vi "Project.vi"() -> ()   [LabVIEW 2026]
doc: "This example performs writes and reads on a serial port, as directed by the user. You can press the Write and Read buttons, and change the Read Count, while the example is running.\n\nThe parameters set for the serial port must match the parameters of the connected instrument or device. In this example, the Read Count parameter specifies the number of bytes that the serial port reads. If there were more bytes at the port than the specified number, those bytes would not be read. If there were less bytes at the port than the specified number, you would receive a timeout error.\n\nThis example expands upon the flow control options for XON and XOFF, allowing the user to choose those control characters. Also, the user can enable or disable a termination character. Some devices require a termination character in order to identify the end of command strings. Some devices send a termination character to signify the end of data to be read. This example shows how you can end the Read operation once a termination character is detected in the buffer and/or append a termination character at the end of the Write data."
uses:
  Serial - Settings.ctl
  Control 1.ctl
  ESP32-PSOC-State Machine-1.ctl
  <vilib>/Instr/_visa.llb/VISA Flush IO Buffer Mask.ctl
  <vilib>/Instr/_visa.llb/VISA Configure Serial Port (Instr).vi
panel:
  in  "HARD START":bool
  in  "INTERMEDIATE START":bool
  out "error":bool
  out "Connected":bool
  out "Serial Settings:Number of Bytes at Serial Port":u32
  out "Processing":string
  in  "EASY START":bool
  in  "IDENTIFY":bool
  in  "CALIBRATE":bool
  in  "Enum":T1
  in  "Termination Character":u8=10 format="%.0x"
  in  "End Write on Termination Character?":bool=TRUE
  in  "EXIT":bool
  out "Read Count":u32=1000
  out "Raw Response":string
  in  "XON/XOFF Characters":T2={"XON"=enum."DC1", "XOFF"=enum."DC3"}
  in  "Serial Settings":T3={"baud rate"=115200, "data bits"=8, "parity"=enum."None", "stop bits"=10, "flow control"=0} {"flow control" items=["None"=0, "XON/XOFF"=1, "RTS/CTS"=2, "DTR/DSR"=4]; "stop bits" items=["1.0"=10, "1.5"=15, "2.0"=20]; "data bits" min=5 max=8 step=1; "baud rate" items=["75"=75, "110"=110, "134"=134, "150"=150, "300"=300, "600"=600, "1200"=1200, "1800"=1800, "2400"=2400, "4800"=4800, "7200"=7200, "9600"=9600, "14400"=14400, "19200"=19200, "28800"=28800, "38400"=38400, "56000"=56000, "57600"=57600, "115200"=115200, "128000"=128000, "230400"=230400]}
  in  "End Read on Termination Character?":bool=TRUE
  in  "Serial Port":refnum<visa-resource-name>="COM4"
  # "What is LabView currently doing?"
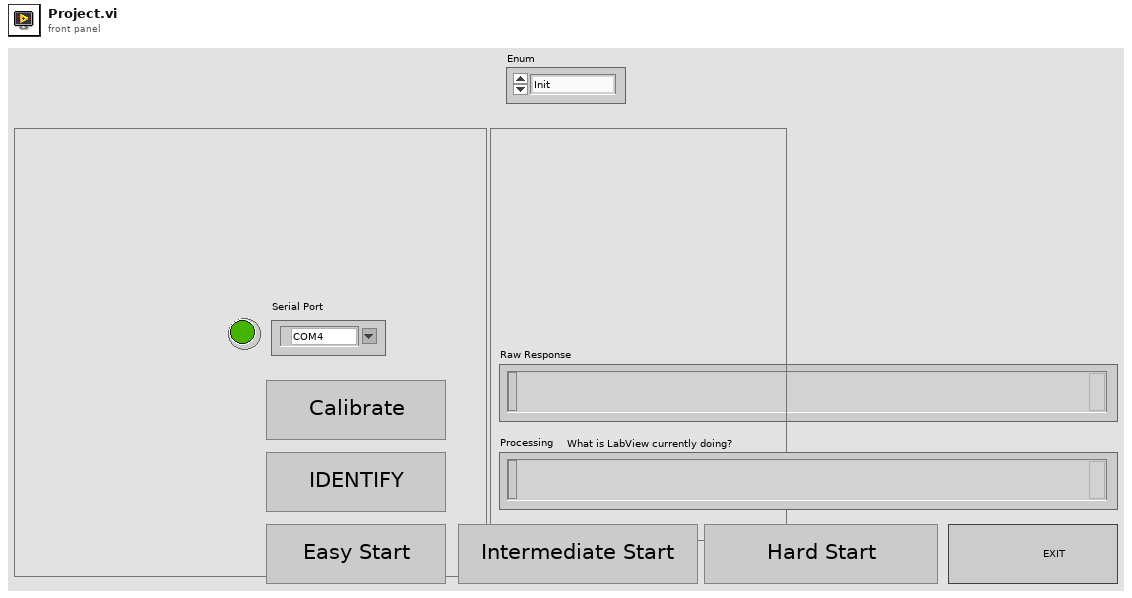
[diagram p1: front panel]
types:
  T1 = typedef "ESP32-PSOC-State Machine-1.ctl" = enum8{"Init", "Connect", "idle", "send", "wait", "receive", "que", "error", "exit"}
  T2 = typedef "Control 1.ctl" = cluster{"XON":enum16{"NUL", "SOH", "STX", "ETX", "EOT", "ENQ", "ACK", "BEL", "BS", "HT", "LF", "VT", "FF", "CR", "SO", "SI", "DLE", "DC1", "DC2", "DC3", "DC4", "NAK", "SYN", "ETB", "CAN", "EM", "SUB", "ESC", "FS", "GS", "RS", "US", "SP", "!", "\"", "#", "$", "%", "&", "'", "(", ")", "*", "+", ",", "- (-)", ".", "/", "0", "1", "2", "3", "4", "5", "6", "7", "8", "9", ":", ";", "<", "=", ">", "?", "@", "A", "B", "C", "D", "E", "F", "G", "H", "I", "J", "K", "L", "M", "N", "O", "P", "Q", "R", "S", "T", "U", "V", "W", "X", "Y", "Z", "[", "\\", "]", "^", "_", "`", "a", "b", "c", "d", "e", "f", "g", "h", "i", "j", "k", "l", "m", "n", "o", "p", "q", "r", "s", "t", "u", "v", "w", "x", "y", "z", "{", "|", "}", "~"}, "XOFF":enum16{"NUL", "SOH", "STX", "ETX", "EOT", "ENQ", "ACK", "BEL", "BS", "HT", "LF", "VT", "FF", "CR", "SO", "SI", "DLE", "DC1", "DC2", "DC3", "DC4", "NAK", "SYN", "ETB", "CAN", "EM", "SUB", "ESC", "FS", "GS", "RS", "US", "SP", "!", "\"", "#", "$", "%", "&", "'", "(", ")", "*", "+", ",", "- (-)", ".", "/", "0", "1", "2", "3", "4", "5", "6", "7", "8", "9", ":", ";", "<", "=", ">", "?", "@", "A", "B", "C", "D", "E", "F", "G", "H", "I", "J", "K", "L", "M", "N", "O", "P", "Q", "R", "S", "T", "U", "V", "W", "X", "Y", "Z", "[", "\\", "]", "^", "_", "`", "a", "b", "c", "d", "e", "f", "g", "h", "i", "j", "k", "l", "m", "n", "o", "p", "q", "r", "s", "t", "u", "v", "w", "x", "y", "z", "{", "|", "}", "~"}}
  T3 = typedef "Serial - Settings.ctl" = cluster{"baud rate":u32, "data bits":u16, "parity":enum16{"None", "Odd", "Even", "Mark", "Space"}, "stop bits":u16, "flow control":u16}
  T4 = enum16{"NUL", "SOH", "STX", "ETX", "EOT", "ENQ", "ACK", "BEL", "BS", "HT", "LF", "VT", "FF", "CR", "SO", "SI", "DLE", "DC1", "DC2", "DC3", "DC4", "NAK", "SYN", "ETB", "CAN", "EM", "SUB", "ESC", "FS", "GS", "RS", "US", "SP", "!", "\"", "#", "$", "%", "&", "'", "(", ")", "*", "+", ",", "- (-)", ".", "/", "0", "1", "2", "3", "4", "5", "6", "7", "8", "9", ":", ";", "<", "=", ">", "?", "@", "A", "B", "C", "D", "E", "F", "G", "H", "I", "J", "K", "L", "M", "N", "O", "P", "Q", "R", "S", "T", "U", "V", "W", "X", "Y", "Z", "[", "\\", "]", "^", "_", "`", "a", "b", "c", "d", "e", "f", "g", "h", "i", "j", "k", "l", "m", "n", "o", "p", "q", "r", "s", "t", "u", "v", "w", "x", "y", "z", "{", "|", "}", "~"}
  T5 = typedef "VISA Flush IO Buffer Mask.ctl" = u16
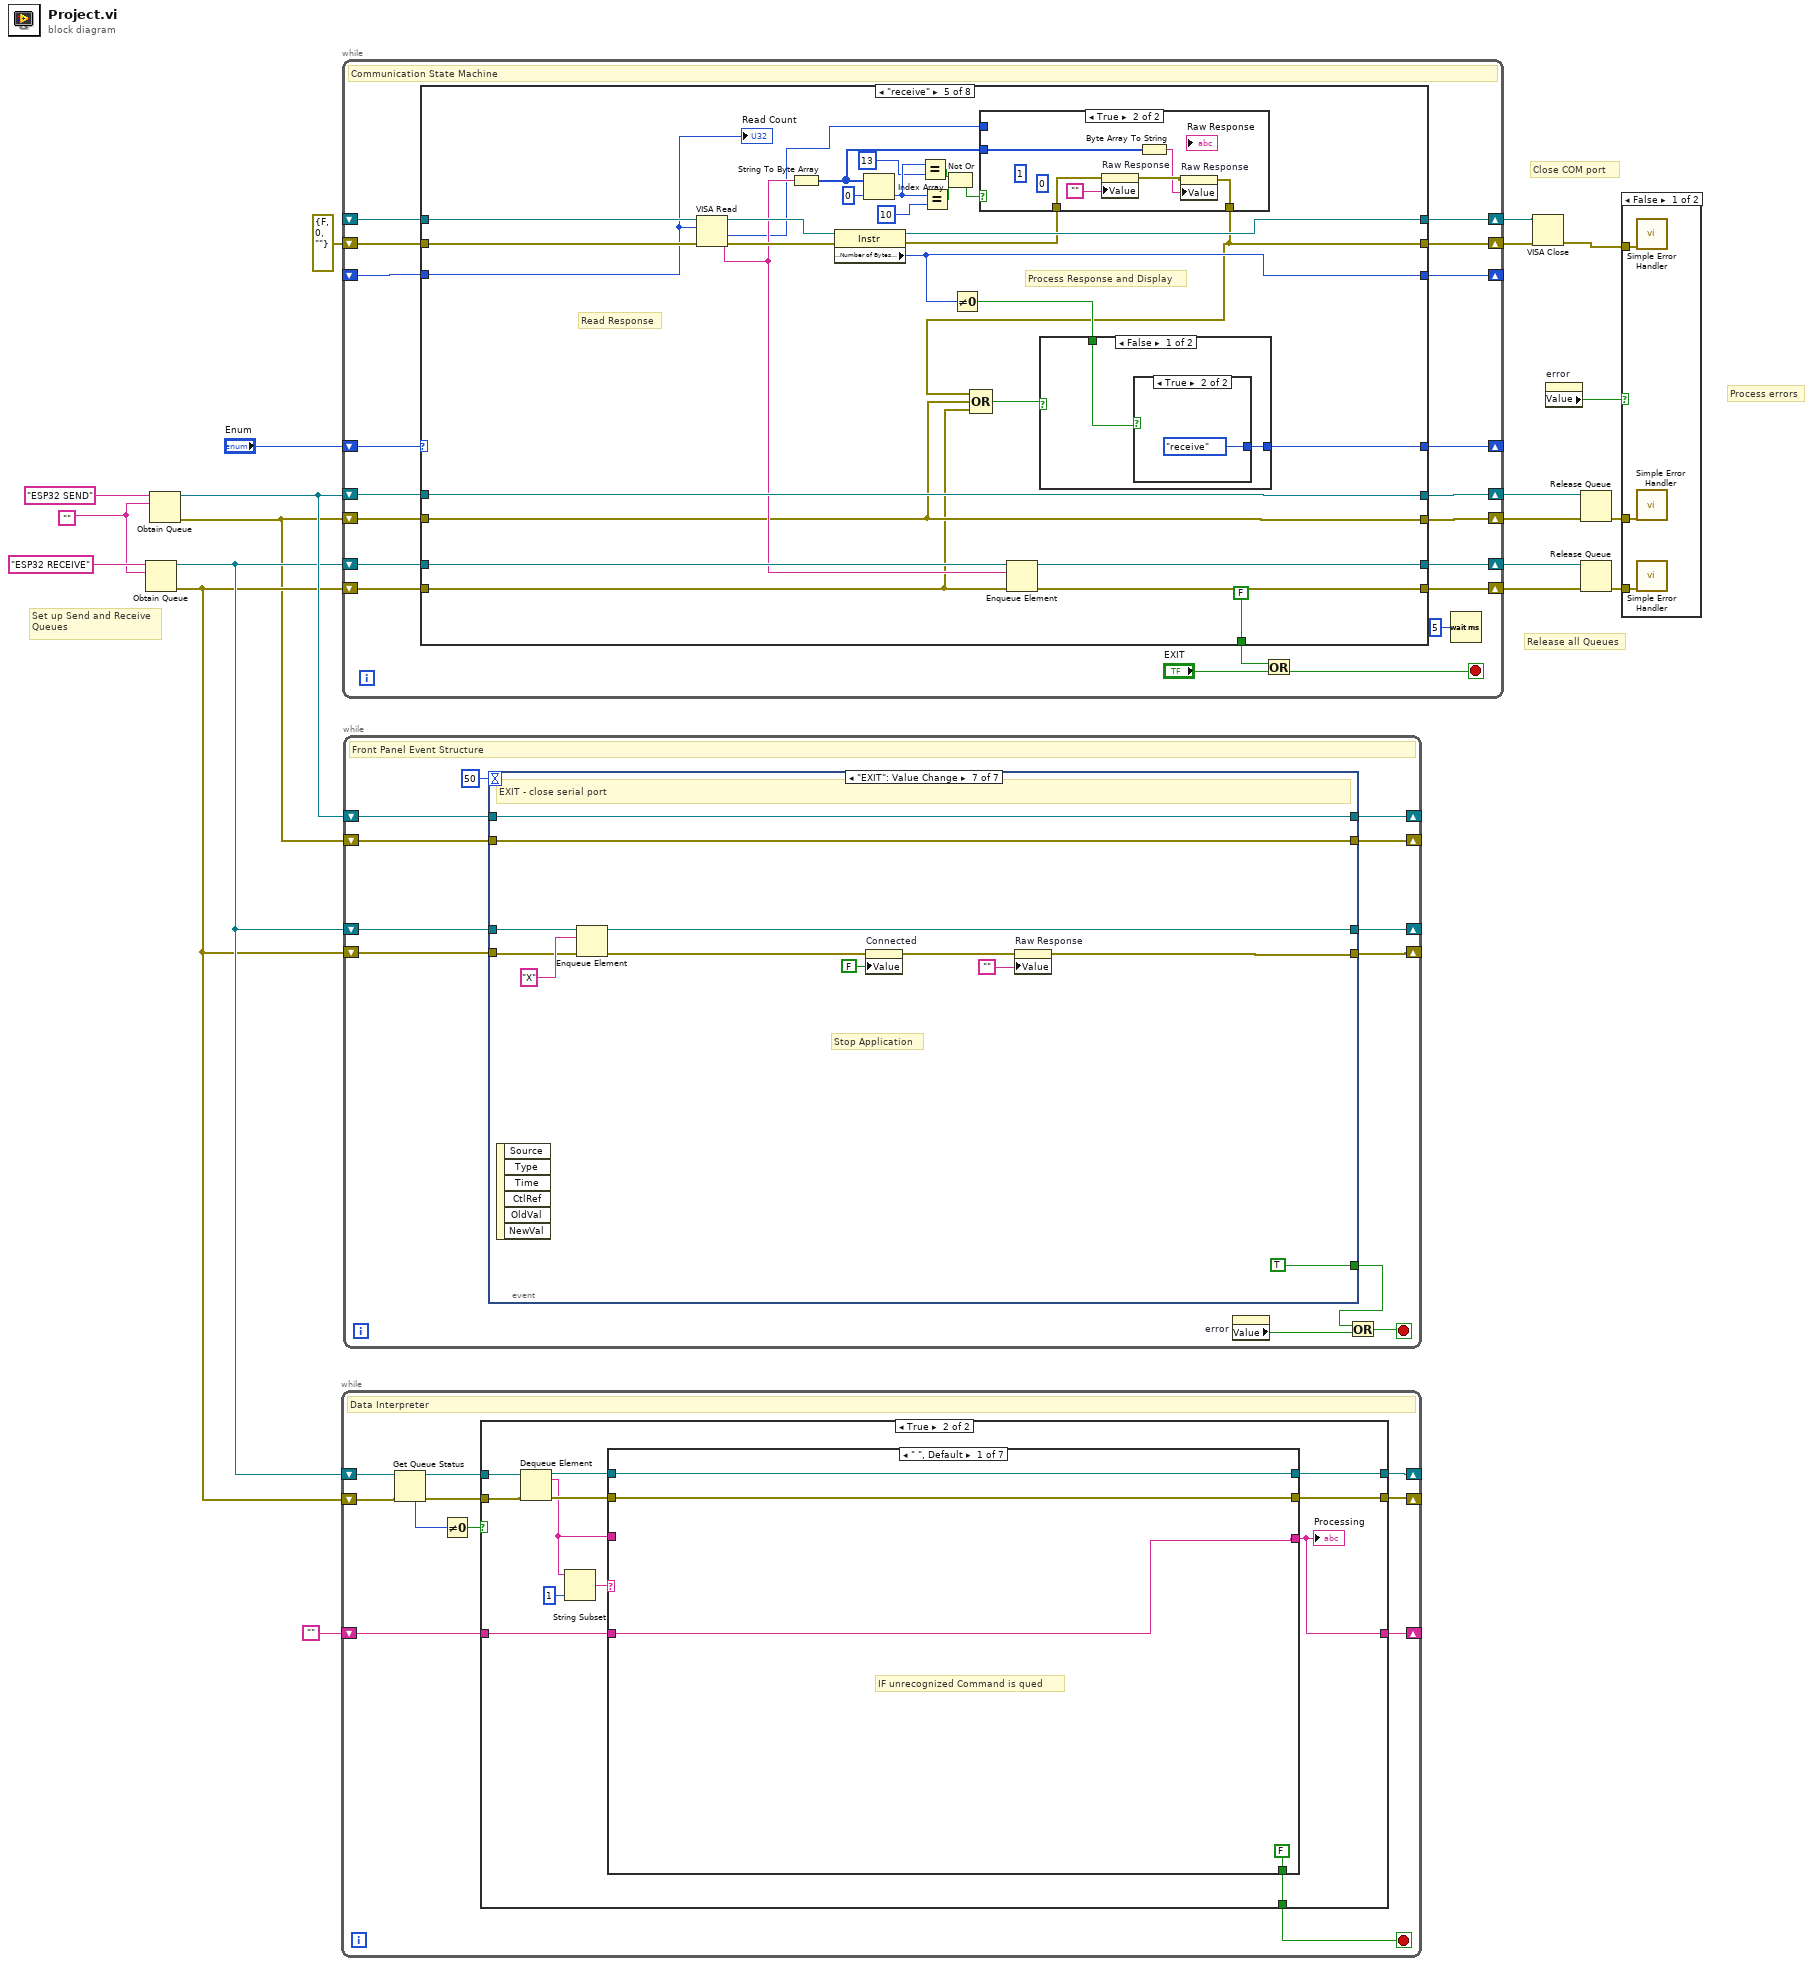
[diagram p0: block diagram]
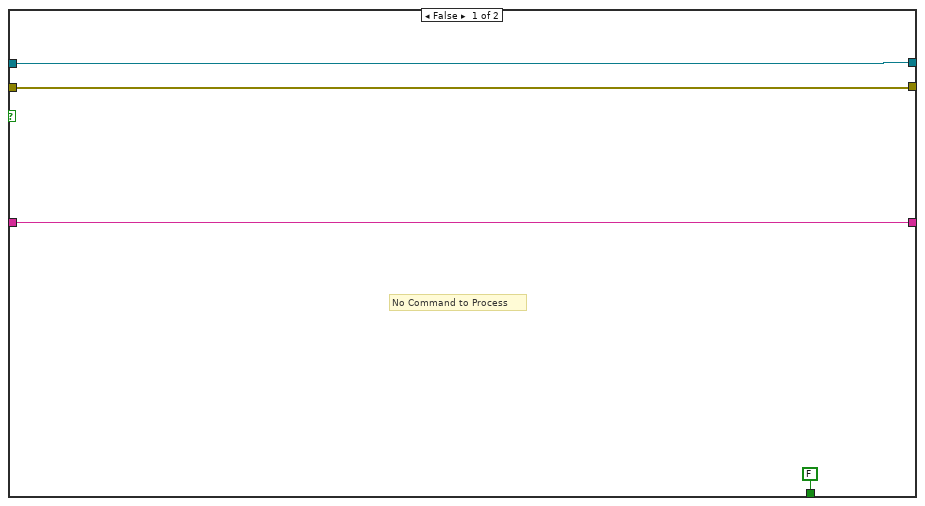
[diagram p3: hidden frame]
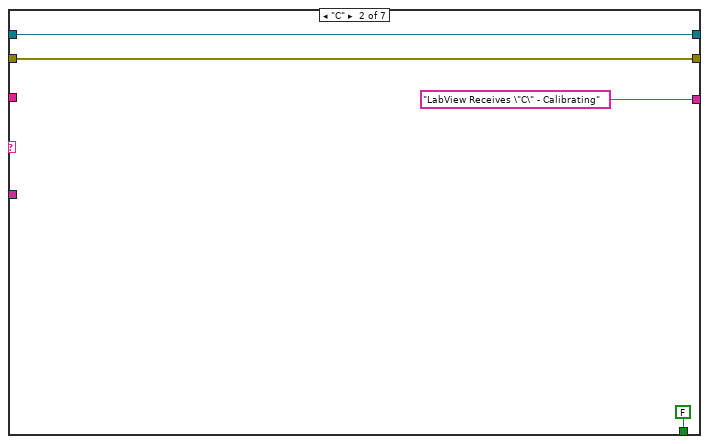
[diagram p4: hidden frame]
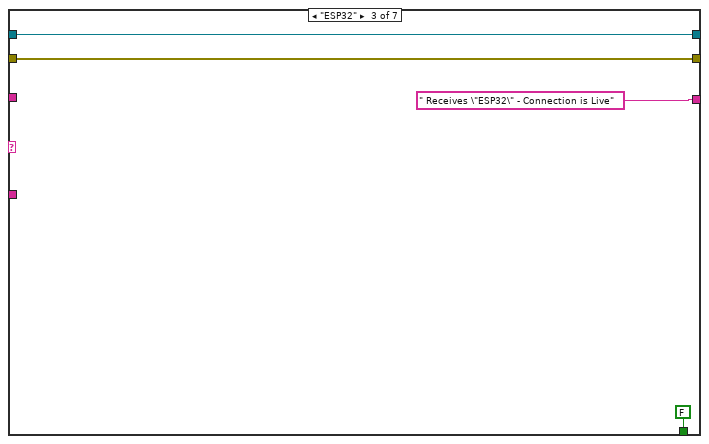
[diagram p5: hidden frame]
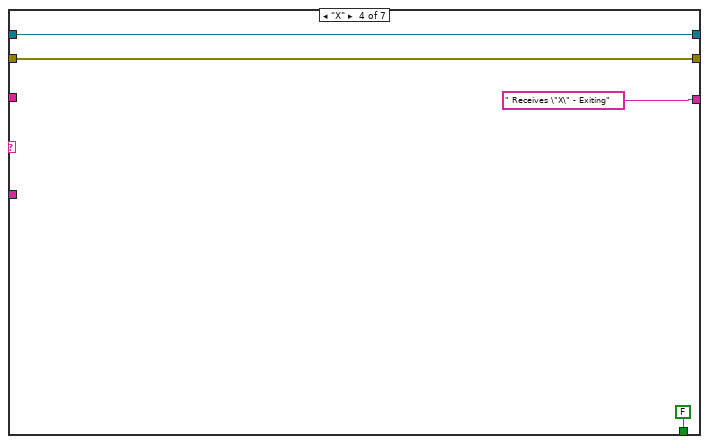
[diagram p6: hidden frame]
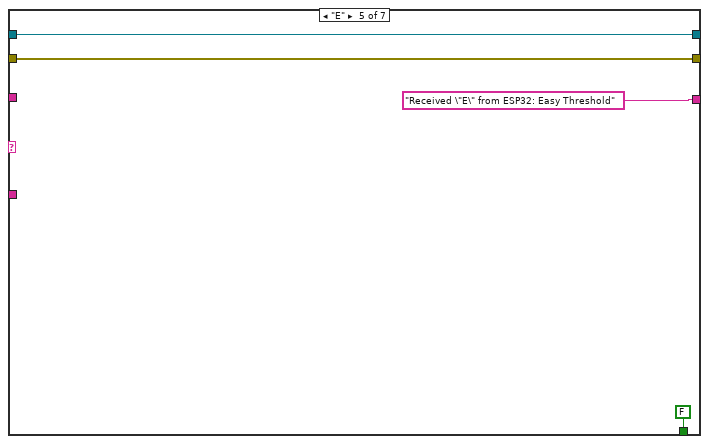
[diagram p7: hidden frame]
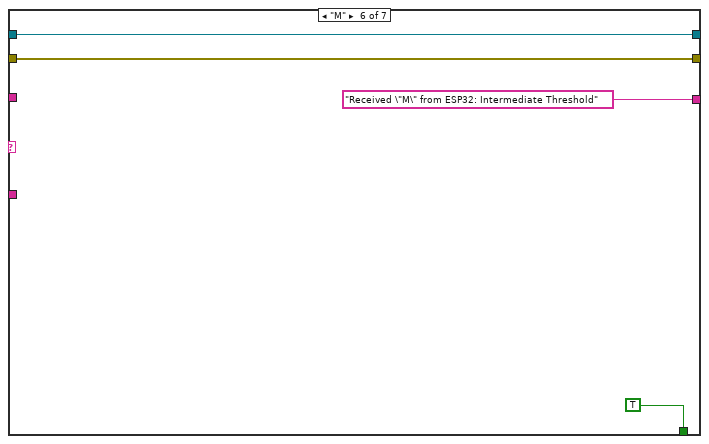
[diagram p8: hidden frame]
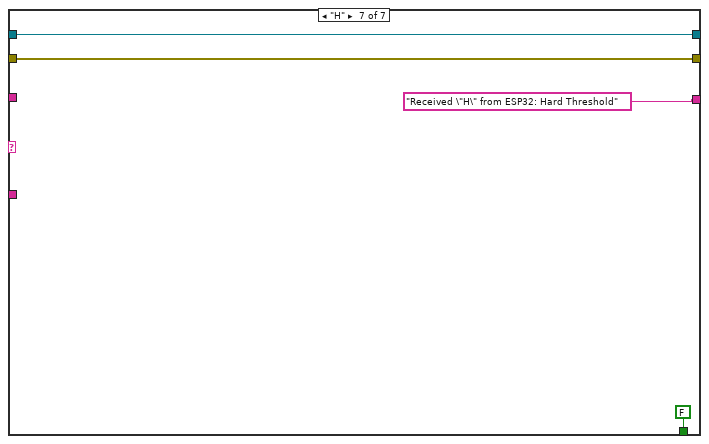
[diagram p9: hidden frame]
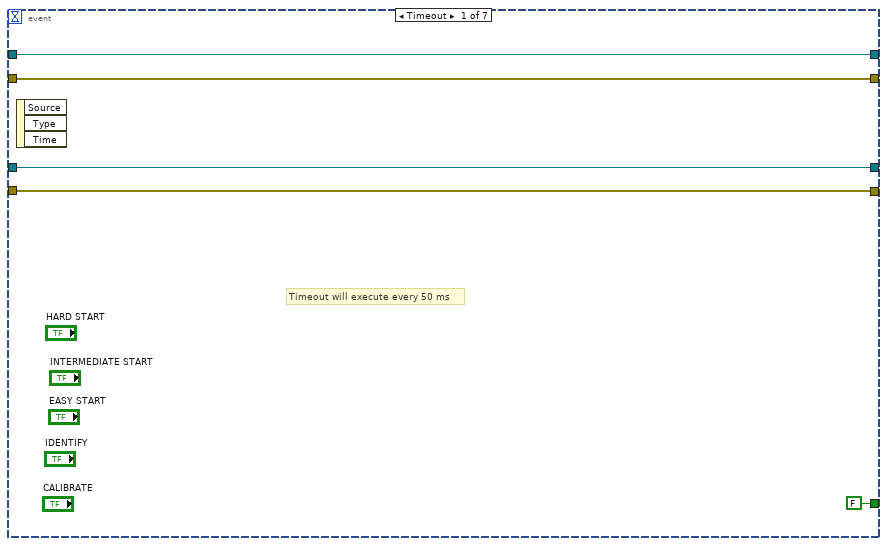
[diagram p10: hidden frame]
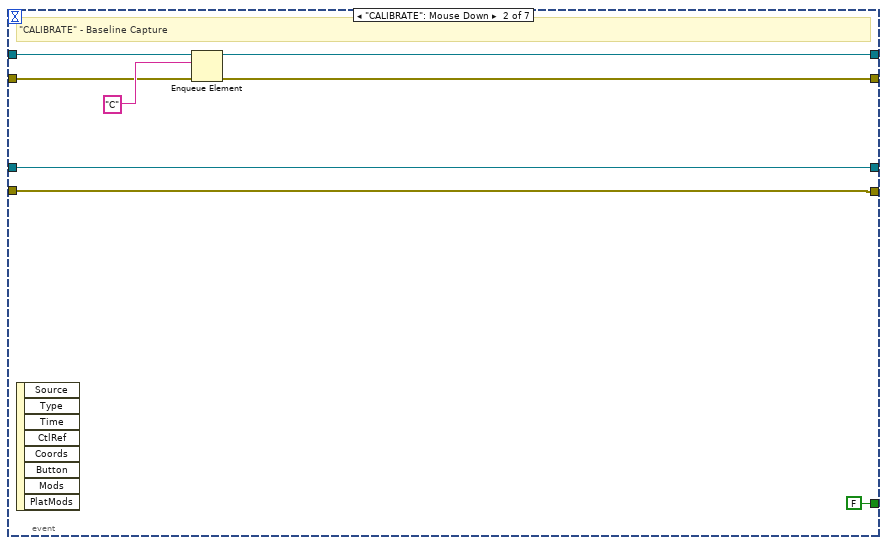
[diagram p11: hidden frame]
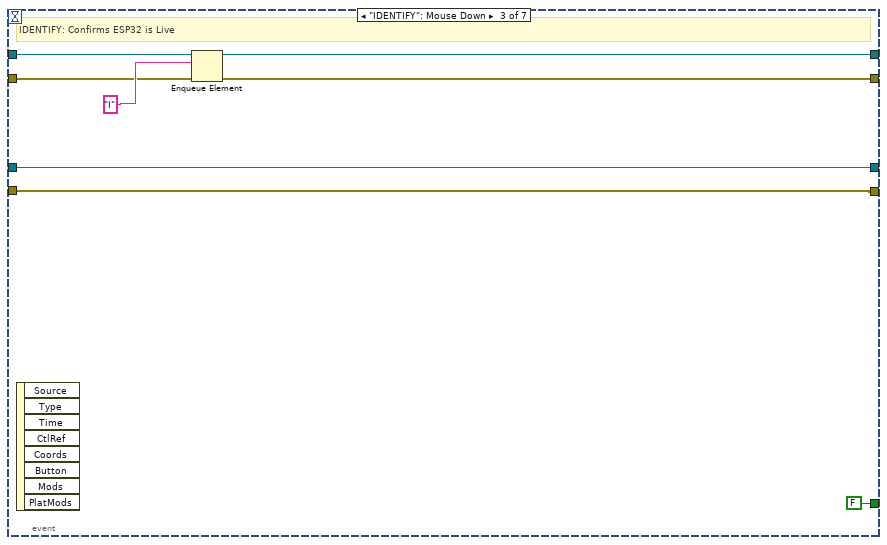
[diagram p12: hidden frame]
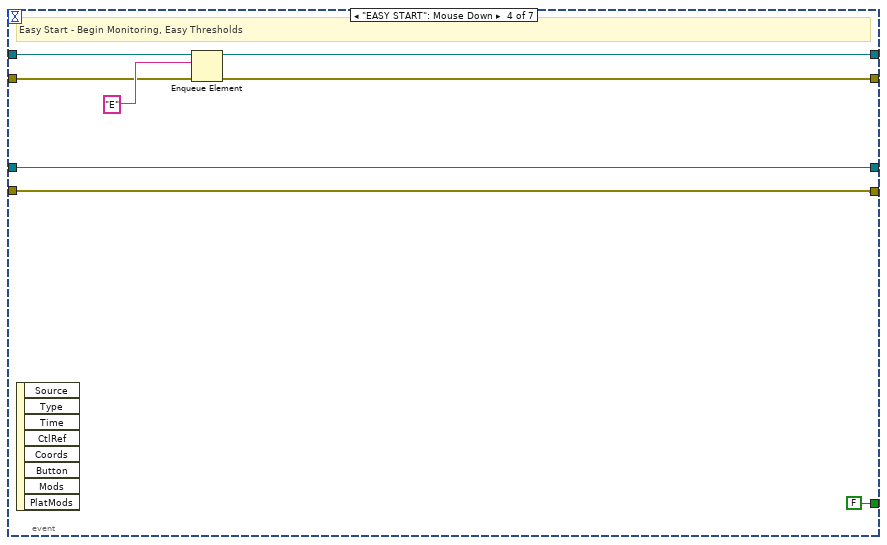
[diagram p13: hidden frame]
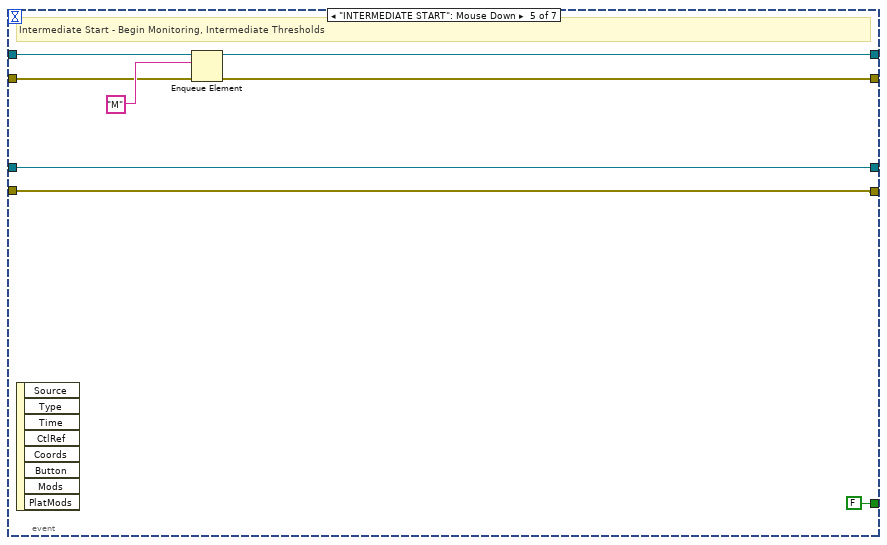
[diagram p14: hidden frame]
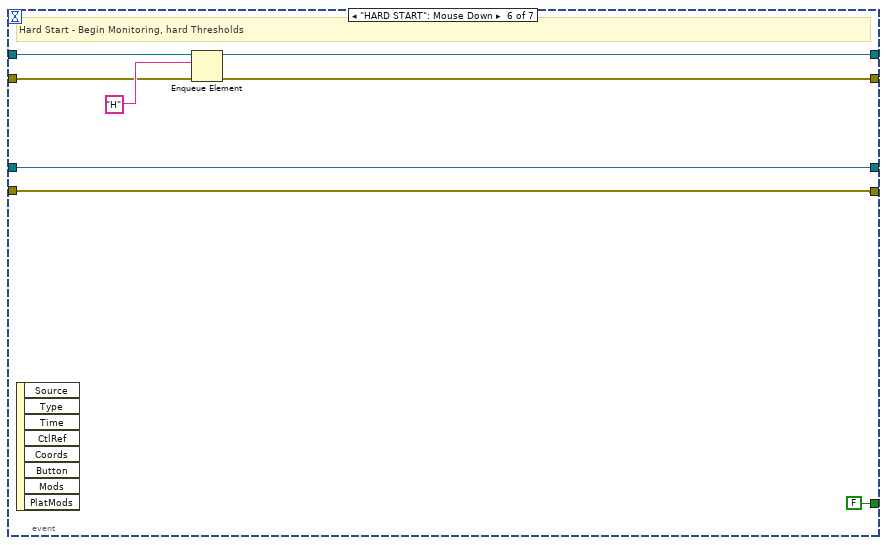
[diagram p15: hidden frame]
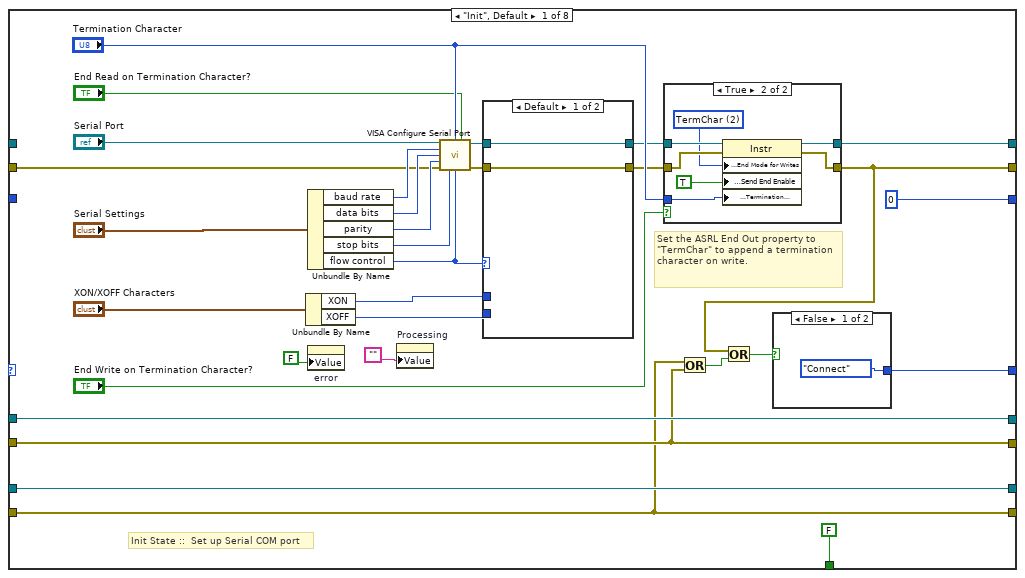
[diagram p16: hidden frame]
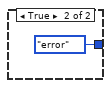
[diagram p17: hidden frame]
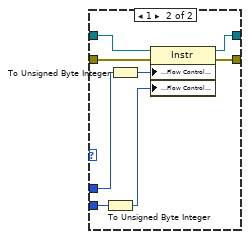
[diagram p19: hidden frame]
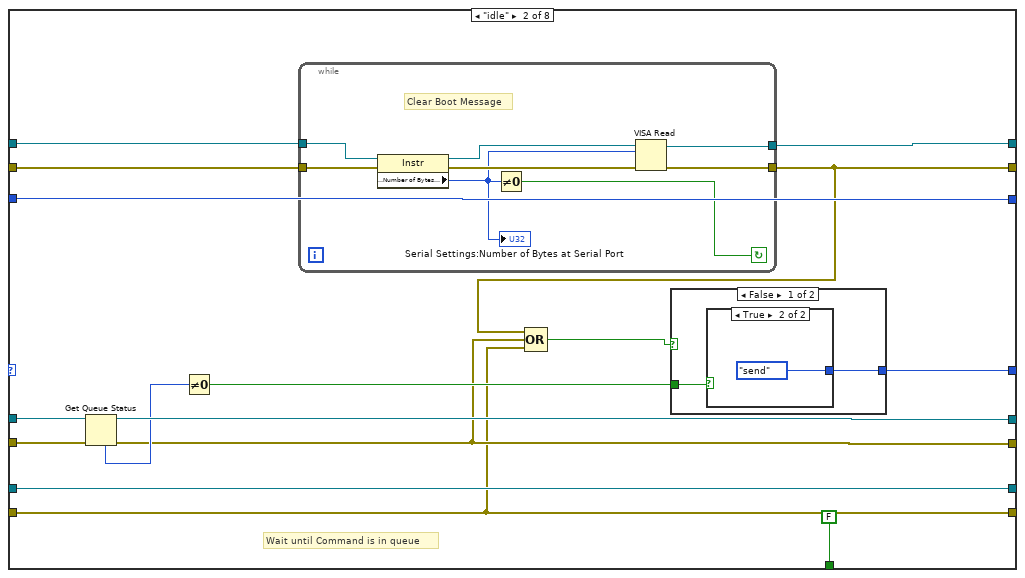
[diagram p20: hidden frame]
diagram:
  w10 = ""
  # "Process errors"
  # "Release all Queues"
  # "Close COM port"
  # "Set up Send and Receive\nQueues"
  n1 = Obtain Queue(name (unnamed)="ESP32 RECEIVE", element data type=w10) -> (queue out=w9:refnum<queue>, error out=w8:errorcluster)  [unwired: 3 in, 1 out]
  n2 = Obtain Queue(name (unnamed)="ESP32 SEND", element data type=w10) -> (queue out=w12:refnum<queue>, error out=w2:errorcluster)  [unwired: 3 in, 1 out]
  n3 = while {
    shift-right: [w25] -> _
    shift-left: w9 -> [w31]
    shift-right: [w24] -> _
    shift-left: w8 -> [w30]
    shift-right: [w22] -> _
    shift-left: "" -> [w21]
    stop <- w23 stop-if-true
    # "Data Interpreter"
    n4 = Get Queue Status(queue=w31, error in (no error)=w30) -> (queue out=w27:refnum<queue>, error out=w26:errorcluster, # elements in queue=w29:i32)  [unwired: 1 in, 5 out]
    n5 = Not Equal To 0?(x=w29) -> (x != 0?=w28:bool)
    n6 = case shown="True" w28 {
      tunnel: w27 -> [w35 w47]
      tunnel: w26 -> [w34 w46]
      tunnel: [w35 w41] -> w25
      tunnel: [w34 w40] -> w24
      tunnel: [FALSE w39] -> w23
      tunnel: [w32 w37] -> w22
      tunnel: w21 -> [w32 w36]
      frame False {
        # "No Command to Process"
      }
      frame True {
        n7 = Dequeue Element(queue=w47, error in (no error)=w46) -> (queue out=w45:refnum<queue>, element=w38:string, error out=w44:errorcluster)  [unwired: 1 in, 1 out]
        n8 = String Subset(string=w38, length (rest)=1 ("length (rest)")) -> (substring=w42:string)  [unwired: 1 in]
        n9 = case shown="\" \", Default" w42 {
          tunnel: w45 -> [w51 w55 w59 w63 w67 w71 w75]
          tunnel: w44 -> [w50 w54 w58 w62 w66 w70 w74]
          tunnel: [w51 w55 w59 w63 w67 w71 w75] -> w41
          tunnel: [w50 w54 w58 w62 w66 w70 w74] -> w40
          tunnel: w38 -> [_ _ _ _ _ _ _]
          tunnel: [FALSE FALSE FALSE FALSE FALSE TRUE FALSE] -> w39
          tunnel: [w48 "LabView Receives \"C\" - Calibrating" " Receives \"ESP32\" - Connection is Live" " Receives \"X\" - Exiting" "Received \"E\" from ESP32: Easy Threshold" "Received \"M\" from ESP32: Intermediate Threshold" "Received \"H\" from ESP32: Hard Threshold"] -> w37
          tunnel: w36 -> [w48 _ _ _ _ _ _]
          frame " ", Default {
            # "IF unrecognized Command is qued"
          }
          frame "C" {
          }
          frame "ESP32" {
          }
          frame "X" {
          }
          frame "E" {
          }
          frame "M" {
          }
          frame "H" {
          }
        }
        "Processing" <- w37
      }
    }
  }
  n10 = while {
    shift-right: [w87] -> w20
    shift-left: w12 -> [w95]
    shift-right: [w86] -> w18
    shift-left: w2 -> [w94]
    shift-right: [w85] -> w19
    shift-left: w9 -> [w93]
    shift-right: [w84] -> w15
    shift-left: w8 -> [w92]
    shift-right: [w79] -> _
    shift-left: "Enum" -> [w78]
    shift-right: [w91] -> w14
    shift-left: _ -> [w88]
    shift-right: [w90] -> w13
    shift-left: errorcluster {"status"=FALSE, "code"=0, "source"=""} ("error out") -> [w89]
    shift-right: [w83] -> _
    shift-left: _ -> [w82]
    stop <- w77 stop-if-true
    # "Communication State Machine"
    n11 = case shown="\"receive\"" w78 {
      selector: w78 -> [_ _ _ _ _ _ w290 _]
      tunnel: [w125 w161 w197 w214 w252 w274 w289 w312] -> w87
      tunnel: [w99 w151 w189 w208 w235 w271 w288 w311] -> w86
      tunnel: [w105 w159 w190 w217 w253 ESP32-PSOC-State_Machine-1."exit" ("Enum") w290 ESP32-PSOC-State_Machine-1."idle" ("Enum")] -> w79
      tunnel: w95 -> [w125 w163 w199 w214 w252 w274 w289 w312]
      tunnel: w94 -> [w99 w162 w198 w208 w235 w271 w288 w311]
      tunnel: w93 -> [w126 w157 w196 w211 w247 w273 w287 w310]
      tunnel: w92 -> [w98 w150 w188 w207 w234 w270 w278 w309]
      tunnel: [w107 w154 w185 w216 w243 w276 w293 w314] -> w91
      tunnel: [w101 w152 w183 w209 w236 w272 w292 w315] -> w90
      tunnel: w89 -> [w103 w153 w193 w215 w238 w272 w292 w316]
      tunnel: w88 -> [_ w155 w195 w205 w250 w276 w293 w317]
      tunnel: [w126 w157 w196 w211 w245 w273 w285 w310] -> w85
      tunnel: [w98 w150 w188 w207 w246 w270 w281 w309] -> w84
      tunnel: [u32 0 ("Bytes at Port") w156 w177 w213 w248 w275 w291 w313] -> w83
      tunnel: w82 -> [_ w156 _ _ w226 w275 w291 w313]
      tunnel: [FALSE FALSE FALSE FALSE FALSE FALSE TRUE FALSE] -> w76
      frame "Init", Default {
        # "Init State ::  Set up Serial COM port"
        # "Set the ASRL End Out property to \"TermChar\" to append a termination character on write."
        n12 = Unbundle By Name("XON/XOFF Characters") -> ("XON"=w119:T4, "XOFF"=w120:T4)
        n13 = Unbundle By Name("Serial Settings") -> ("baud rate"=w115:u32, "data bits"=w114:u16, "parity"=w113:enum16{"None", "Odd", "Even", "Mark", "Space"}, "stop bits"=w112:u16, "flow control"=w118:u16)
        n14 = property on="error" class="Bool (strict)"("Value"=FALSE ("error")) -> ()  [unwired: 2 in, 2 out]
        n15 = property on="Processing" class="Str"("Value"="") -> ()  [unwired: 2 in, 2 out]
        n16 = call-poly "VISA Configure Serial Port"("VISA resource name"="Serial Port", "termination char\n(0xA = '\\n' = LF)"="Termination Character", "Enable Termination\nChar (T)"="End Read on Termination Character?", "baud rate (9600)"=w115, "data bits (8)"=w114, "parity (0:none)"=w113, "error in (no error)"=w103, "stop bits (10: 1 bit)"=w112, "flow control (0:none)"=w118) -> ("VISA resource name out"=w111:refnum<visa-resource-name>, "error out"=w110:errorcluster)  [unwired: 1 in, 4 out]
        n17 = case shown="Default" w118 {
          tunnel: [w138 w147] -> w121
          tunnel: [w139 w146] -> w122
          tunnel: w110 -> [w138 w145]
          tunnel: w111 -> [w139 w144]
          tunnel: w119 -> [_ w143]
          tunnel: w120 -> [_ w142]
          frame Default {
          }
          frame 1 {
            n18 = To Unsigned Byte Integer(number=w142) -> (unsigned 8bit integer=w141:u8)
            n19 = To Unsigned Byte Integer(number=w143) -> (unsigned 8bit integer=w140:u8)
            n20 = property class="Instr"(reference=w144, error in=w145, "Serial Settings:Flow Control XON Character"=w140, "Serial Settings:Flow Control XOFF Character"=w141) -> (reference out=w146:refnum<visa-resource-name>, error out=w147:errorcluster)
          }
        }
        n21 = case shown="True" "End Write on Termination Character?" {
          tunnel: w122 -> [w129 w137]
          tunnel: w121 -> [w130 w136]
          tunnel: [w129 w135] -> w107
          tunnel: [w130 w134] -> w101
          tunnel: "Termination Character" -> [_ w132]
          frame False {
          }
          frame True {
            w133 = u16 2 items=["None", "LastBit", "TermChar", "Break"] ("Serial Settings:Serial End Mode for Writes")
            n22 = property class="Instr"(reference=w137, error in=w136, "Serial Settings:End Mode for Writes"=w133, "Message Based Settings:Send End Enable"=TRUE, "Message Based Settings:Termination Character"=w132) -> (reference out=w135:refnum<visa-resource-name>, error out=w134:errorcluster)
          }
        }
        n23 = Or(x=w98, y=w99) -> (x .or. y?=w100:bool)
        n24 = Or(x=w101, y=w100) -> (x .or. y?=w102:bool)
        n25 = case shown="False" w102 {
          tunnel: [ESP32-PSOC-State_Machine-1."Connect" ("Enum") ESP32-PSOC-State_Machine-1."error" ("Enum")] -> w105
          frame False {
          }
          frame True {
          }
        }
      }
      frame "idle" {
        # "Wait until Command is in queue"
        n26 = Get Queue Status(queue=w163, error in (no error)=w162) -> (queue out=w161:refnum<queue>, error out=w151:errorcluster, # elements in queue=w160:i32)  [unwired: 1 in, 5 out]
        n27 = Not Equal To 0?(x=w160) -> (x != 0?=w158:bool)
        n28 = while {
          tunnel: w155 -> [w176]
          tunnel: [w172] -> w154
          tunnel: w153 -> [w175]
          tunnel: [w170] -> w152
          stop <- w174 continue-if-true
          # "Clear Boot Message"
          n29 = property class="Instr"(reference=w176, error in=w175) -> (reference out=w173:refnum<visa-resource-name>, error out=w171:errorcluster, "Serial Settings:Number of Bytes at Serial Port"=w169:u32)
          "Serial Settings:Number of Bytes at Serial Port" <- w169
          n30 = Not Equal To 0?(x=w169) -> (x != 0?=w174:bool)
          n31 = VISA Read(VISA resource name=w173, byte count=w169, error in (no error)=w171) -> (VISA resource name out=w172:refnum<visa-resource-name>, error out=w170:errorcluster)  [unwired: 2 out]
        }
        n32 = Compound Arithmetic op=OR(w152, w151, w150) -> (w149:bool)
        n33 = case shown="False" w149 {
          tunnel: [w165 ESP32-PSOC-State_Machine-1."error" ("Enum")] -> w159
          tunnel: w158 -> [w164 _]
          frame False {
            n34 = case shown="True" w164 {
              tunnel: [ESP32-PSOC-State_Machine-1."idle" ("Enum") ESP32-PSOC-State_Machine-1."send" ("Enum")] -> w165
              frame False {
              }
              frame True {
              }
            }
          }
          frame True {
          }
        }
      }
      frame "send" {
        w191 = T5 64 items=["Flush Receive Buffer"=16, "Write Transmit Buffer to Device"=32, "Flush Receive Buffer (No I/O)"=64, "Flush Transmit Buffer"=128] ("Mask")
        # "Read and Discard Echo Command"
        # "Wait for Response"
        # "Send Command"
        n35 = Dequeue Element(queue=w199, error in (no error)=w198) -> (queue out=w197:refnum<queue>, element=w181:string, error out=w189:errorcluster)  [unwired: 1 in, 1 out]
        n36 = VISA Flush I/O Buffer(VISA resource name=w195, mask (16)=w191, error in (no error)=w193) -> (VISA resource name out=w194:refnum<visa-resource-name>, error out=w192:errorcluster)
        n37 = Concatenate Strings(w181, "\r\n") -> (w180:string)
        n38 = VISA Write(VISA resource name=w194, write buffer=w180, error in (no error)=w192) -> (VISA resource name out=w179:refnum<visa-resource-name>, error out=w184:errorcluster)  [unwired: 1 out]
        n39 = flat-sequence {
          tunnel: w179 -> [w201]
          tunnel: [w201] -> w178
          frame #0 {
            n40 = Wait (ms)(milliseconds to wait=u32 15) -> ()  [unwired: 1 out]
          }
        }
        n41 = property class="Instr"(reference=w178, error in=w184) -> (reference out=w185:refnum<visa-resource-name>, error out=w183:errorcluster, "Serial Settings:Number of Bytes at Serial Port"=w177:u32)
        n42 = Compound Arithmetic op=OR(w183, w189, w188) -> (w187:bool)
        n43 = case shown="False" w187 {
          tunnel: [ESP32-PSOC-State_Machine-1."wait" ("Enum") ESP32-PSOC-State_Machine-1."error" ("Enum")] -> w190
          frame False {
          }
          frame True {
          }
        }
      }
      frame "wait" {
        # "Wait for actual Response"
        n44 = flat-sequence {
          tunnel: w205 -> [w219]
          tunnel: [w219] -> w204
          frame #0 {
            n45 = Wait (ms)(milliseconds to wait=u32 15) -> ()  [unwired: 1 out]
          }
        }
        n46 = property class="Instr"(reference=w204, error in=w215) -> (reference out=w216:refnum<visa-resource-name>, error out=w209:errorcluster, "Serial Settings:Number of Bytes at Serial Port"=w213:u32)
        n47 = Not Equal To 0?(x=w213) -> (x != 0?=w212:bool)
        n48 = Compound Arithmetic op=OR(w209, w208, w207) -> (w210:bool)
        n49 = case shown="False" w210 {
          tunnel: [w221 ESP32-PSOC-State_Machine-1."error" ("Enum")] -> w217
          tunnel: w212 -> [w220 _]
          frame False {
            n50 = case shown="True" w220 {
              tunnel: [ESP32-PSOC-State_Machine-1."wait" ("Enum") ESP32-PSOC-State_Machine-1."receive" ("Enum")] -> w221
              frame False {
              }
              frame True {
              }
            }
          }
          frame True {
          }
        }
      }
      frame "receive" {
        # "Process Response and Display"
        # "Read Response"
        n51 = VISA Read(VISA resource name=w250, byte count=w226, error in (no error)=w238) -> (VISA resource name out=w244:refnum<visa-resource-name>, read buffer=w240:string, return count=w225:u32, error out=w249:errorcluster)
        n52 = String To Byte Array(string=w240) -> (unsigned byte array=w239:u8[])
        n53 = property class="Instr"(reference=w244, error in=w249) -> (reference out=w243:refnum<visa-resource-name>, error out=w237:errorcluster, "Serial Settings:Number of Bytes at Serial Port"=w248:u32)
        n54 = Index Array(array=w239, index=0) -> (element=w231:u8)
        n55 = Equal?(x=w231, y=u8 13) -> (x = y?=w229:bool)
        n56 = Equal?(x=w231, y=u8 10) -> (x = y?=w228:bool)
        n57 = Not Or(1:w228, 2:w229) -> (0:w227:bool)
        n58 = Not Equal To 0?(x=w248) -> (x != 0?=w251:bool)
        n59 = case shown="True" w227 {
          tunnel: w239 -> [_ w260]
          tunnel: w237 -> [w259 w262]
          tunnel: [w259 w261] -> w236
          tunnel: w225 -> [_ _]
          frame False {
          }
          frame True {
            (unwired) 1 ("length")
            (unwired) 0 ("index")
            n60 = property on="Raw Response" class="Str"(error in=w262, "Value"="") -> (error out=w264:errorcluster)  [unwired: 1 in, 1 out]
            n61 = Byte Array To String(unsigned byte array=w260) -> (string=w263:string)
            n62 = property on="Raw Response" class="Str"(error in=w264, "Value"=w263) -> (error out=w261:errorcluster)  [unwired: 1 in, 1 out]
          }
        }
        n63 = Compound Arithmetic op=OR(w236, w235, w234) -> (w233:bool)
        n64 = Enqueue Element(queue=w247, element=w240, error in (no error)=w234) -> (queue out=w245:refnum<queue>, error out=w246:errorcluster)  [unwired: 1 in, 1 out]
        n65 = case shown="False" w233 {
          tunnel: [w255 ESP32-PSOC-State_Machine-1."error" ("Enum")] -> w253
          tunnel: w251 -> [w254 _]
          frame False {
            n66 = case shown="True" w254 {
              tunnel: [ESP32-PSOC-State_Machine-1."idle" ("Enum") ESP32-PSOC-State_Machine-1."receive" ("Enum")] -> w255
              frame False {
              }
              frame True {
              }
            }
          }
          frame True {
          }
        }
        "Read Count" <- w226
      }
      frame "error" {
        # "Process any error"
        n67 = Build Array(w272, w271, w270) -> (w269:errorcluster[])
        n68 = for {
          tunnel: w269 -> [w277] mode=indexing
          n69 = call <vilib>:"General Error Handler.vi"("error in (no error)"=w277) -> ()  [unwired: 10 in, 5 out]
        }
        "error" <- TRUE ("error")
      }
      frame "exit" {
        # "Exit due to error"
        n70 = Enqueue Element(queue=w287, element="S", error in (no error)=w278) -> (queue out=w285:refnum<queue>, error out=w283:errorcluster)  [unwired: 1 in, 1 out]
        n71 = property on="Connected" class="Bool (strict)"(error in=w283, "Value"=FALSE ("Connected")) -> (error out=w282:errorcluster)  [unwired: 1 in, 1 out]
        n72 = property on="Raw Response" class="Str"(error in=w282, "Value"="") -> (error out=w281:errorcluster)  [unwired: 1 in, 1 out]
      }
      frame "Connect" {
        # "Validating connection"
        # "Send ID to validate connection"
        # "Clear any residual characters"
        n73 = while {
          shift-right: [w341] -> w305
          shift-left: w316 -> [w347]
          shift-right: [w340] -> w306
          shift-left: w317 -> [w346]
          stop <- w345 continue-if-true
          n74 = property class="Instr"(reference=w346, error in=w347) -> (reference out=w343:refnum<visa-resource-name>, error out=w342:errorcluster, "Bytes at Port"=w339:u32)
          n75 = VISA Read(VISA resource name=w343, byte count=w339, error in (no error)=w342) -> (VISA resource name out=w340:refnum<visa-resource-name>, read buffer=w338:string, error out=w341:errorcluster)  [unwired: 1 out]
          n76 = Wait (ms)(milliseconds to wait=u32 5) -> ()  [unwired: 1 out]
          n77 = Search/Split String(string=w338, search string/char (-)="Commands") -> (match + rest of string=w336:string)  [unwired: 1 in, 2 out]
          n78 = String Length(string=w336) -> (length=w335:i32)
          n79 = Equal To 0?(x=w335) -> (x = 0?=w345:bool)
        }
        n80 = Concatenate Strings("I" ("write buffer"), "\r\n") -> (w294:string)
        n81 = VISA Write(VISA resource name=w306, write buffer=w294, error in (no error)=w305) -> (VISA resource name out=w300:refnum<visa-resource-name>, error out=w304:errorcluster)  [unwired: 1 out]
        n82 = flat-sequence {
          tunnel: w300 -> [w334]
          tunnel: [w334] -> w299
          frame #0 {
            n83 = Wait (ms)(milliseconds to wait=u32 5) -> ()  [unwired: 1 out]
          }
        }
        n84 = property class="Instr"(reference=w299, error in=w304) -> (reference out=w302:refnum<visa-resource-name>, error out=w303:errorcluster, "Bytes at Port"=w301:u32)
        n85 = VISA Read(VISA resource name=w302, byte count=w301, error in (no error)=w303) -> (VISA resource name out=w297:refnum<visa-resource-name>, error out=w298:errorcluster)  [unwired: 2 out]
        n86 = while {
          shift-right: [w321] -> w315
          shift-left: w298 -> [w327]
          shift-right: [w322] -> w314
          shift-left: w297 -> [w320]
          stop <- w318 stop-if-true
          n87 = flat-sequence {
            tunnel: w320 -> [w332]
            tunnel: [w332] -> w319
            frame #0 {
              n88 = Wait (ms)(milliseconds to wait=u32 15) -> ()  [unwired: 1 out]
            }
          }
          n89 = property class="Instr"(reference=w319, error in=w327) -> (reference out=w325:refnum<visa-resource-name>, error out=w326:errorcluster, "Bytes at Port"=w324:u32)
          n90 = VISA Read(VISA resource name=w325, byte count=w324, error in (no error)=w326) -> (VISA resource name out=w322:refnum<visa-resource-name>, read buffer=w323:string, error out=w321:errorcluster)  [unwired: 1 out]
          n91 = Search/Split String(string=w323, search string/char (-)="ESP32") -> (match + rest of string=w329:string)  [unwired: 1 in, 2 out]
          n92 = String Length(string=w329) -> (length=w328:i32)
          n93 = Not Equal To 0?(x=w328) -> (x != 0?=w318:bool)
          "Connected" <- w318
        }
      }
    }
    n94 = Or(x=w76, y="EXIT") -> (x .or. y?=w77:bool)
    n95 = Wait (ms)(milliseconds to wait=u32 5) -> ()  [unwired: 1 out]
  }
  n96 = while {
    shift-right: [w356] -> _
    shift-left: w12 -> [w357]
    shift-right: [w355] -> _
    shift-left: w2 -> [w358]
    shift-right: [w351] -> _
    shift-left: w9 -> [w354]
    shift-right: [w352] -> _
    shift-left: w8 -> [w353]
    stop <- w348 stop-if-true
    # "Front Panel Event Structure"
    n97 = event shown="[6] \"EXIT\": Value Change" {
      selector: _ -> [_ _ _ _ _ _ _]
      dyn-events: _ -> [_ _ _ _ _ _ _]
      timeout: 50 -> [_ _ _ _ _ _ _]
      tunnel: w358 -> [w363 w370 w378 w386 w394 w402 w414]
      tunnel: w357 -> [w360 w372 w380 w388 w396 w404 w415]
      tunnel: [w360 w369 w377 w385 w393 w401 w415] -> w356
      tunnel: [w363 w368 w376 w384 w392 w400 w414] -> w355
      tunnel: [FALSE FALSE FALSE FALSE FALSE FALSE TRUE] -> w350
      tunnel: w354 -> [w362 w366 w374 w382 w390 w398 w413]
      tunnel: w353 -> [w361 w365 w373 w381 w389 w397 w411]
      tunnel: [w361 w365 w373 w381 w389 w397 w406] -> w352
      tunnel: [w362 w366 w374 w382 w390 w398 w410] -> w351
      event Timeout {
        # "Timeout will execute every 50 ms"
        n98 = event-data() -> ()  [unwired: 1 in, 3 out]
      }
      event "CALIBRATE": Mouse Down {
        # "\"CALIBRATE\" - Baseline Capture"
        n99 = event-data() -> ()  [unwired: 1 in, 8 out]
        n100 = Enqueue Element(queue=w372, element="C", error in (no error)=w370) -> (queue out=w369:refnum<queue>, error out=w368:errorcluster)  [unwired: 1 in, 1 out]
      }
      event "IDENTIFY": Mouse Down {
        # "IDENTIFY: Confirms ESP32 is Live"
        n101 = event-data() -> ()  [unwired: 1 in, 8 out]
        n102 = Enqueue Element(queue=w380, element="I", error in (no error)=w378) -> (queue out=w377:refnum<queue>, error out=w376:errorcluster)  [unwired: 1 in, 1 out]
      }
      event "EASY START": Mouse Down {
        # "Easy Start - Begin Monitoring, Easy Thresholds"
        n103 = event-data() -> ()  [unwired: 1 in, 8 out]
        n104 = Enqueue Element(queue=w388, element="E", error in (no error)=w386) -> (queue out=w385:refnum<queue>, error out=w384:errorcluster)  [unwired: 1 in, 1 out]
      }
      event "INTERMEDIATE START": Mouse Down {
        # "Intermediate Start - Begin Monitoring, Intermediate Thresholds"
        n105 = event-data() -> ()  [unwired: 1 in, 8 out]
        n106 = Enqueue Element(queue=w396, element="M", error in (no error)=w394) -> (queue out=w393:refnum<queue>, error out=w392:errorcluster)  [unwired: 1 in, 1 out]
      }
      event "HARD START": Mouse Down {
        # "Hard Start - Begin Monitoring, hard Thresholds"
        n107 = event-data() -> ()  [unwired: 1 in, 8 out]
        n108 = Enqueue Element(queue=w404, element="H", error in (no error)=w402) -> (queue out=w401:refnum<queue>, error out=w400:errorcluster)  [unwired: 1 in, 1 out]
      }
      event "EXIT": Value Change {
        # "Stop Application"
        # "EXIT - close serial port"
        n109 = event-data() -> ()  [unwired: 1 in, 6 out]
        n110 = Enqueue Element(queue=w413, element="X", error in (no error)=w411) -> (queue out=w410:refnum<queue>, error out=w409:errorcluster)  [unwired: 1 in, 1 out]
        n111 = property on="Connected" class="Bool (strict)"(error in=w409, "Value"=FALSE ("Connected")) -> (error out=w407:errorcluster)  [unwired: 1 in, 1 out]
        n112 = property on="Raw Response" class="Str"(error in=w407, "Value"="") -> (error out=w406:errorcluster)  [unwired: 1 in, 1 out]
      }
    }
    n113 = property on="error" class="Bool (strict)"() -> ("Value"=w349:bool)  [unwired: 2 in, 2 out]
    n114 = Or(x=w350, y=w349) -> (x .or. y?=w348:bool)
  }
  n115 = VISA Close(VISA resource name=w14, error in (no error)=w13) -> (error out=w5:errorcluster)
  n116 = property on="error" class="Bool (strict)"() -> ("Value"=w1:bool)  [unwired: 2 in, 2 out]
  n117 = Release Queue(queue=w20, error in (no error)=w18) -> (error out=w4:errorcluster)  [unwired: 1 in, 2 out]
  n118 = Release Queue(queue=w19, error in (no error)=w15) -> (error out=w3:errorcluster)  [unwired: 1 in, 2 out]
  n119 = case shown="False" w1 {
    tunnel: w5 -> [w419 _]
    tunnel: w4 -> [w418 _]
    tunnel: w3 -> [w417 _]
    frame False {
      n120 = call <vilib>:"Simple Error Handler.vi"("error in (no error)"=w419) -> ()  [unwired: 1 in, 8 out]
      n121 = call <vilib>:"Simple Error Handler.vi"("error in (no error)"=w418) -> ()  [unwired: 1 in, 8 out]
      n122 = call <vilib>:"Simple Error Handler.vi"("error in (no error)"=w417) -> ()  [unwired: 1 in, 8 out]
    }
    frame True {
    }
  }
